vi "ZMC Get Zlib Global Define.vi"(8 "error in (no error)":errorcluster caption="错误输入（无错误）", 9 "buffsize":u32, 10 "pbuffer":string, 11 "pfilenameZlb":string) -> (0 "error out":errorcluster caption="错误输出", 2 "pbuffer out":string, 3 "function return":i32)   [LabVIEW 2015, in "zauxdll.lvlib"]
doc: "int32 __stdcall ZMC_GetZlibGlobalDefine(const char* pfilenameZlb, char* pbuffer, uint32 buffsize);"
uses:
  zauxdll.lvlib
  zmotion.dll
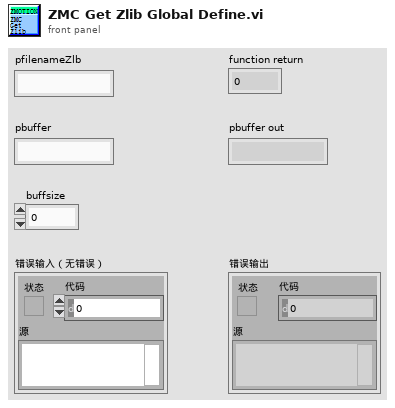
[diagram p1: front panel]
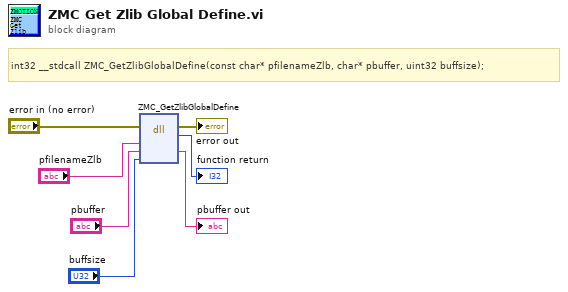
[diagram p0: block diagram]
diagram:
  # "int32 __stdcall ZMC_GetZlibGlobalDefine(const char* pfilenameZlb, char* pbuffer, uint32 buffsize);"
  n1 = dll-call lib="C:/Users/VIC/Desktop/GOGORO_SA/system/LLB/zmotion/zaux/zmotion.*" fn="ZMC_GetZlibGlobalDefine"(error in="error in (no error)", "pfilenameZlb"="pfilenameZlb", "pbuffer"="pbuffer", "buffsize"="buffsize") -> (error out=→"error out":errorcluster, →"function return":i32, "pbuffer"=→"pbuffer out":string)  [unwired: 4 in, 1 out]
